vi "Lab2_batsound.vi"() -> ()   [LabVIEW 2010]
uses:
  <vilib>/sound2/lvsound2.llb/Sound File Read Open.vi
  <vilib>/sound2/lvsound2.llb/Sound File Read (DBL).vi
  <vilib>/measure/maspectr.llb/FFT Spectrum (Mag-Phase) for N Chan.vi
  <vilib>/measure/NI_MAPro.lvlib
panel:
  out "FFT":cluster{"f0":dbl, "df":dbl, "magnitude":dbl[]}[](graph)
  out "Waveform Graph":waveform(dbl)[](graph)
  in  "Path":path
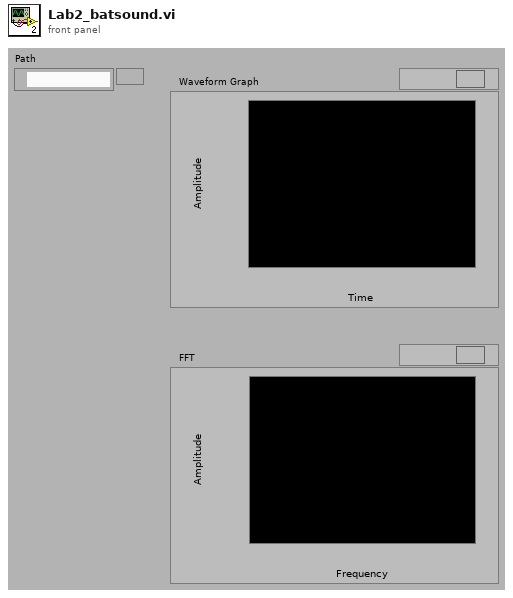
[diagram p1: front panel]
types:
  T1 = typedef "Sound File Refnum.ctl" = refnum<file>
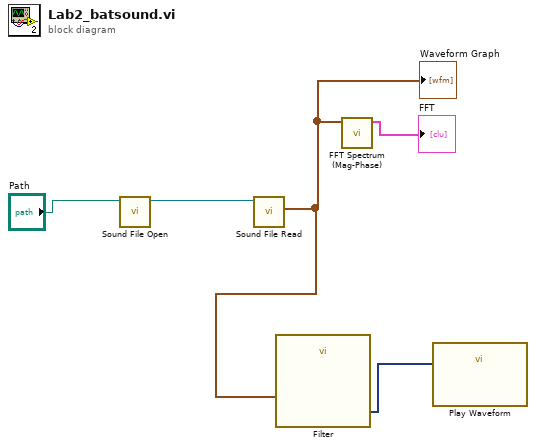
[diagram p0: block diagram]
diagram:
  n1 = call-poly <vilib>:"Sound File Open.vi"("path"="Path") -> ("sound file refnum"=w4:T1)  [unwired: 9 in, 1 out]
  n2 = call-poly <vilib>:"Sound File Read.vi"("sound file refnum"=w4) -> ("data"=w1:waveform(dbl)[])  [unwired: 6 in, 4 out]
  "Waveform Graph" <- w1
  n3 = call "Filter"("Signal"=w1) -> ("Filtered Signal"=w3:dynamicdata)  [unwired: 9 in, 1 out]
  n4 = call-poly <vilib>:"FFT Spectrum (Mag-Phase).vi"("time signals"=w1) -> ("magnitudes"=→"FFT":cluster{"f0":dbl, "df":dbl, "magnitude":dbl[]}[])  [unwired: 6 in, 4 out]
  n5 = call "Play Waveform"("Data"=w3) -> ()  [unwired: 18 in, 1 out]
